vi "Obtener_Posicion_Presionada.vi"(1 "Tablero":cluster{"img":u16, " Btn_Tablero":bool}[][](array[cluster])) -> (0 "Posicion_Presionada":string)   [LabVIEW 2019]
doc: "Permite saber en que posicion del tablero hizo clic el usuario."
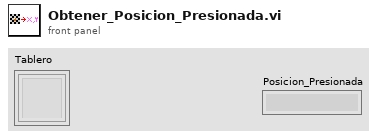
[diagram p1: front panel]
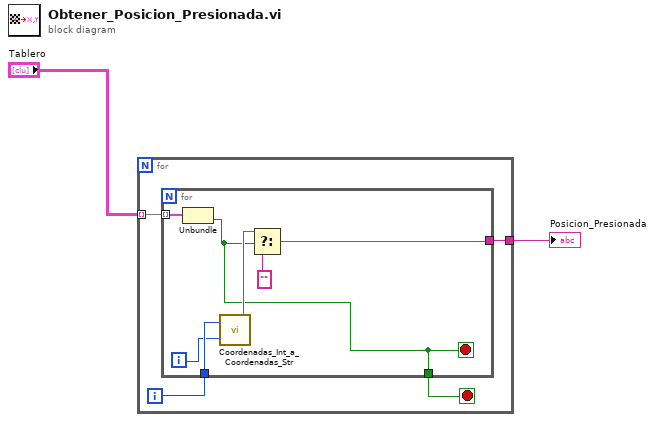
[diagram p0: block diagram]
diagram:
  n1 = for {
    tunnel: [w5] -> w2
    tunnel: "Tablero" -> [w4] mode=indexing
    i -> [w6]
    stop <- w3 stop-if-true
    n2 = for {
      tunnel: w6 -> [w13]
      tunnel: [w9] -> w5
      tunnel: [w7] -> w3
      tunnel: w4 -> [w8] mode=indexing
      i -> [w12]
      stop <- w7 stop-if-true
      n3 = Unbundle(w8) -> ("Btn_Tablero"=w7:bool)  [unwired: 1 out]
      n4 = call "Coordenadas_Int_a_Coordenadas_Str.vi"("Columna"=w12, "Fila"=w13) -> ("Posicion_str"=w11:string)
      n5 = Select(t=w11, s=w7, f="") -> (s? t:f=w9:string)
    }
  }
  "Posicion_Presionada" <- w2
